vi "Test_EmptyList_RetrieveNothing.vi"(8 "error in (no error)":errorcluster, 11 "TestCase in":refnum<class "TestStringList.lvclass">) -> (0 "error out":errorcluster, 3 "TestCase out":refnum<class "TestStringList.lvclass">)   [LabVIEW 2015, in "TestStringList.lvclass"]
uses:
  TestStringList.lvclass
  <vilib>/addons/_JKI Toolkits/VI Tester/TestCase.llb/TestCase.lvclass
  StringList.lvclass
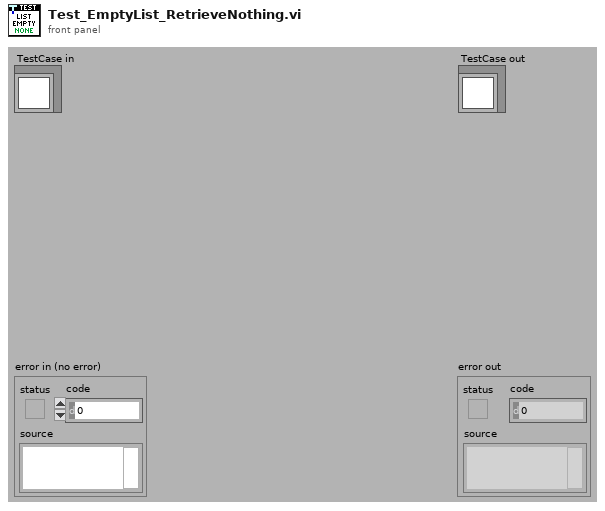
[diagram p1: front panel]
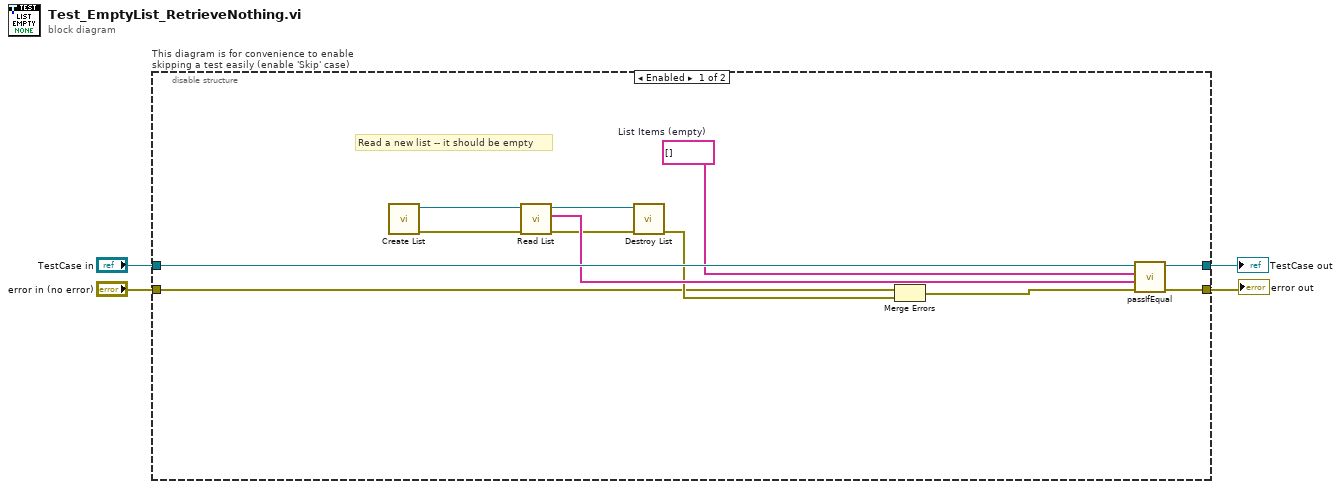
[diagram p0: block diagram]
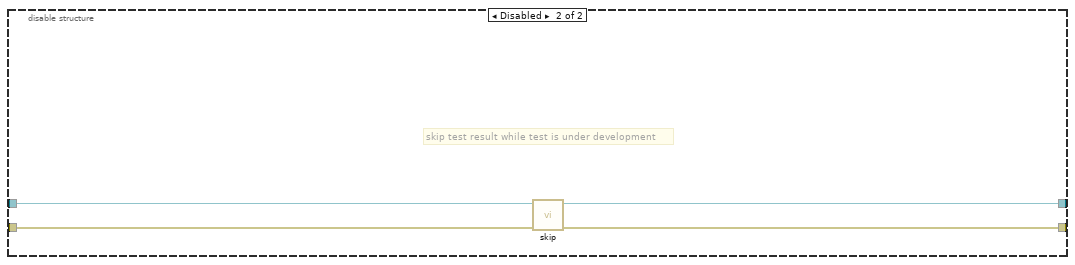
[diagram p2: hidden frame]
diagram:
  n1 = disable-structure "This diagram is for convenience to enable skipping a test easily (enable 'Skip' case)" shown="Enabled" {
    disable-tunnel: "TestCase in" -> [w16 w20]
    disable-tunnel: [w15 w18] -> w1
    disable-tunnel: [w14 w19] -> w3
    disable-tunnel: "error in (no error)" -> [w5 w17]
    frame Enabled {
      w12 = string[] []  # List Items (empty)
      # "Read a new list -- it should be empty"
      n2 = call "Create List.vi"() -> ("error out"=w9:errorcluster, "StringList Reference"=w11:refnum<data-value>)  [unwired: 10 in]
      n3 = call "Read List.vi"("error in (no error)"=w9, "StringList Reference"=w11) -> ("error out"=w8:errorcluster, "Items"=w13:string[], "StringList Reference"=w10:refnum<data-value>)  [unwired: 7 in]
      n4 = call "Destroy List.vi"("error in (no error)"=w8, "StringList Reference"=w10) -> ("error out"=w6:errorcluster)  [unwired: 8 in, 1 out]
      n5 = Merge Errors(w5, w6) -> (w7:errorcluster)
      n6 = call-dynamic "passIfEqual.vi"("error in (no error)"=w7, "y"=w13, "x"=w12, "TestCase in"=w16) -> ("error out"=w14:errorcluster, "TestCase out"=w15:refnum<class "TestStringList.lvclass">)  [unwired: 6 in]
    }
    frame Disabled {
      # "skip test result while test is under development"
      n7 = call <vilib>:"skip.vi"("error in (no error)"=w17, "TestCase in"=w20) -> ("error out"=w19:errorcluster, "TestCase out"=w18:refnum<class "TestStringList.lvclass">)  [unwired: 8 in]
    }
  }
  "error out" <- w3
  "TestCase out" <- w1
